vi "niRFSysCalReader Core.vi"(4 "Enable Interpolation?":bool, 6 "Power (dBm)":dbl, 7 "Frequency (Hz)":dbl, 8 "error in":errorcluster, 9 "niRFSysCalReader State":T1, 10 "Pathloss (dB)":dbl, 11 "niRFSysCalReader Handle":T2) -> (0 "error out":errorcluster, 2 "Pathloss (dB)":dbl, 3 "niRFSysCalReader Handle out":T2)   [LabVIEW 2016, in "niRFSysCalReader.lvlib"]
doc: "Core component of the niRFSysCalReader library."
uses:
  niRFSysCalReader.lvlib
  _INCLUDES/niRFSysCalReader Handle.ctl
  _INCLUDES/niRFSysCalReader Core States.ctl
  <vilib>/Utility/error.llb/Error Cluster From Error Code.vi
  <vilib>/ErrorRing/Error Ring.xnode
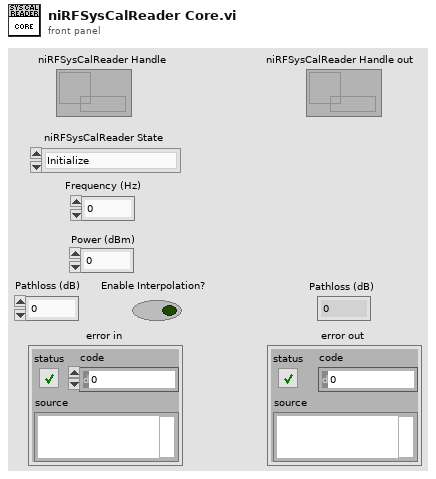
[diagram p1: front panel]
types:
  T1 = typedef "niRFSysCalReader.lvlib/niRFSysCalReader Core States.ctl" = enum16{"Initialize", "Interpolator State", "Add Pathloss", "Get Pathloss", "Remove Pathloss", "Close"}
  T2 = typedef "niRFSysCalReader.lvlib/niRFSysCalReader Handle.ctl" = refnum<data-value>
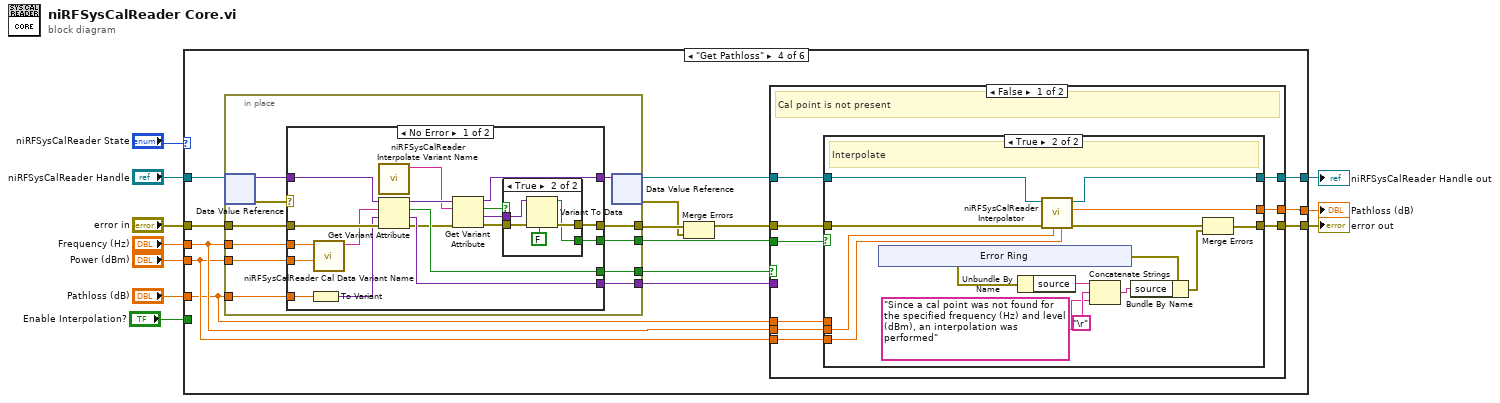
[diagram p0: block diagram]
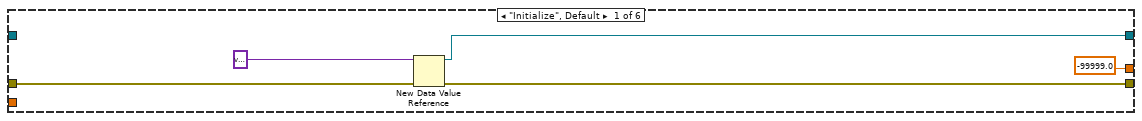
[diagram p2: hidden frame]
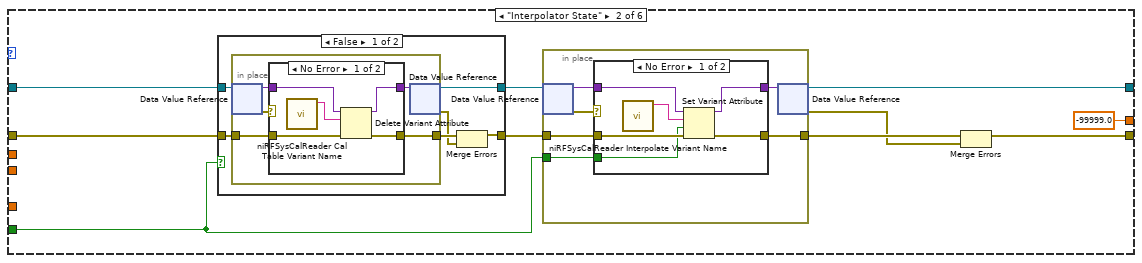
[diagram p3: hidden frame]
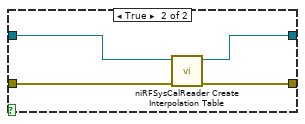
[diagram p5: hidden frame]
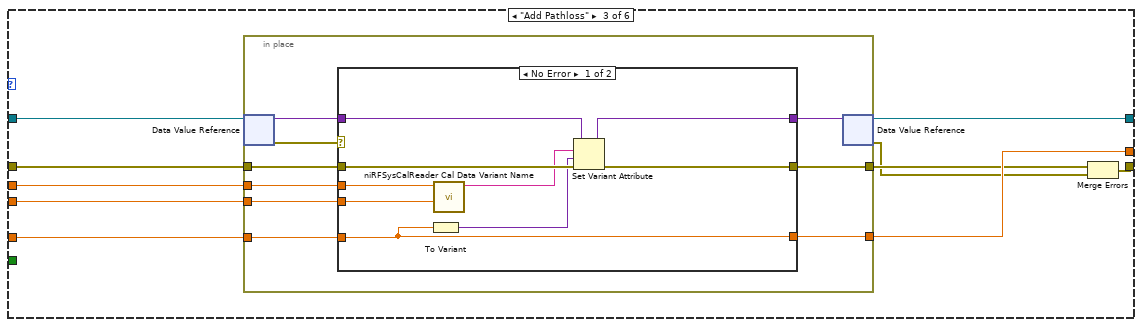
[diagram p7: hidden frame]
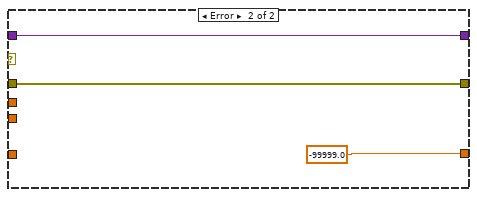
[diagram p8: hidden frame]
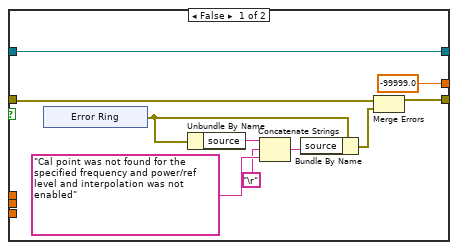
[diagram p9: hidden frame]
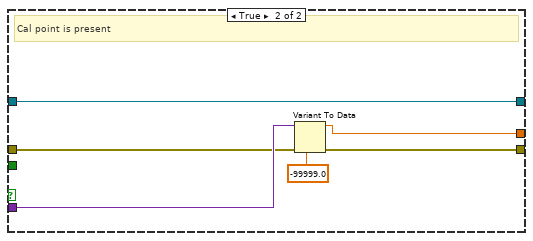
[diagram p10: hidden frame]
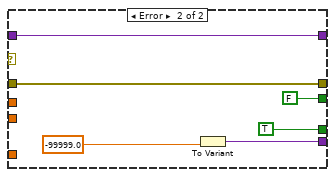
[diagram p12: hidden frame]
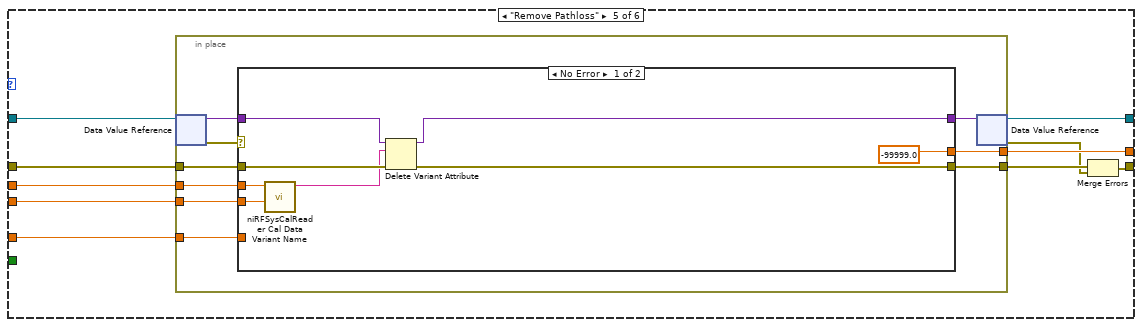
[diagram p13: hidden frame]
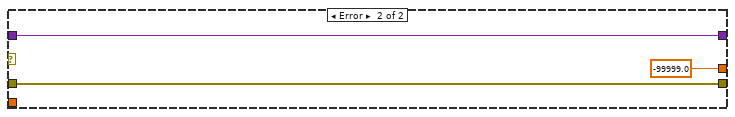
[diagram p14: hidden frame]
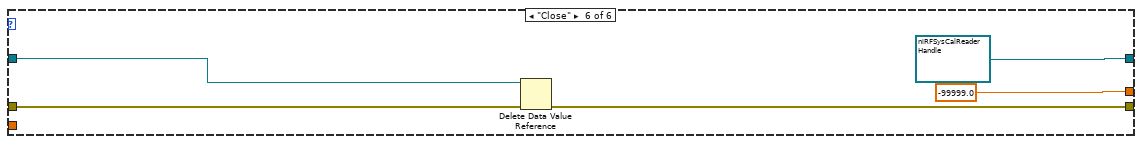
[diagram p15: hidden frame]
diagram:
  n1 = case shown="\"Get Pathloss\"" "niRFSysCalReader State" {
    tunnel: [w14 w25 w69 w97 w204 T2 refnum ("Cal Storage Handle in")] -> w3
    tunnel: [w13 w24 w68 w100 w203 w229] -> w2
    tunnel: "error in" -> [w12 w20 w70 w106 w205 w230]
    tunnel: "niRFSysCalReader Handle" -> [_ w22 w71 w107 w206 w231]
    tunnel: "Frequency (Hz)" -> [_ _ w67 w96 w202 _]
    tunnel: "Power (dBm)" -> [_ _ w66 w95 w201 _]
    tunnel: "Pathloss (dB)" -> [_ _ w65 w94 w200 _]
    tunnel: [-99999.0 -99999.0 ("Interpolated Pathloss (dB)") w64 w99 w199 -99999.0] -> w4
    tunnel: "Enable Interpolation?" -> [_ w16 _ _ _ _]
    frame "Initialize", Default {
      n2 = New Data Value Reference(data value=variant, error in=w12) -> (data value reference=w14:refnum<data-value>, error out=w13:errorcluster)
    }
    frame "Interpolator State" {
      n3 = case shown="False" w16 {
        tunnel: w22 -> [w31 w47]
        tunnel: [w30 w46] -> w21
        tunnel: w20 -> [w29 w45]
        tunnel: [w28 w44] -> w19
        frame False {
          n4 = in-place {
            in-place-border: w29 -> [w34]
            in-place-border: [w33] -> w27
            n5 = in-place-dvr #1(w31) -> (w36:variant, w32:errorcluster)
            n6 = case shown="No Error" w32 {
              tunnel: w36 -> [w41 w43]
              tunnel: [w40 w43] -> w35
              tunnel: w34 -> [w39 w42]
              tunnel: [w38 w42] -> w33
              frame No Error {
                n7 = call "niRFSysCalReader Cal Table Variant Name.vi"() -> ("Calibration Table Name"=w37:string)  [unwired: 11 in]
                n8 = Delete Variant Attribute(4:w39, 6:w37, 7:w41) -> (0:w38:errorcluster, 3:w40:variant)  [unwired: 1 out]
              }
              frame Error {
              }
            }
            n9 = in-place-dvr #1(w35) -> (w30:T2, w26:errorcluster)
          }
          n10 = Merge Errors(w27, w26) -> (w28:errorcluster)
        }
        frame True {
          n11 = call "niRFSysCalReader Create Interpolation Table.vi"("error in"=w45, "niRFSysCalReader Handle"=w47) -> ("error out"=w44:errorcluster, "niRFSysCalReader Handle out"=w46:T2)  [unwired: 7 in, 1 out]
        }
      }
      n12 = in-place {
        in-place-border: [w52] -> w18
        in-place-border: w19 -> [w50]
        in-place-border: w16 -> [w48]
        n13 = in-place-dvr #2(w21) -> (w53:variant, w49:errorcluster)
        n14 = case shown="No Error" w49 {
          tunnel: w53 -> [w59 w61]
          tunnel: [w57 w60] -> w52
          tunnel: [w56 w61] -> w51
          tunnel: w50 -> [w55 w60]
          tunnel: w48 -> [w54 _]
          frame No Error {
            n15 = call "niRFSysCalReader Interpolate Variant Name.vi"() -> ("Interpolation State Name"=w58:string)  [unwired: 11 in]
            n16 = Set Variant Attribute(Variant=w59, name=w58, value=w54, error in=w55) -> (Variant out=w56:variant, error out=w57:errorcluster)  [unwired: 1 out]
          }
          frame Error {
          }
        }
        n17 = in-place-dvr #2(w51) -> (w25:T2, w17:errorcluster)
      }
      n18 = Merge Errors(w18, w17) -> (w24:errorcluster)
    }
    frame "Add Pathloss" {
      n19 = in-place {
        in-place-border: w70 -> [w79]
        in-place-border: [w76] -> w63
        in-place-border: w67 -> [w75]
        in-place-border: w66 -> [w74]
        in-place-border: w65 -> [w73]
        in-place-border: [w72] -> w64
        n20 = in-place-dvr #3(w71) -> (w78:variant, w80:errorcluster)
        n21 = case shown="No Error" w80 {
          tunnel: w79 -> [w89 w91]
          tunnel: w78 -> [w84 w92]
          tunnel: [w83 w92] -> w77
          tunnel: [w88 w91] -> w76
          tunnel: w75 -> [w87 _]
          tunnel: w74 -> [w86 _]
          tunnel: w73 -> [w81 _]
          tunnel: [w81 -99999.0] -> w72
          frame No Error {
            n22 = To Variant(anything=w81) -> (Variant=w82:variant)
            n23 = call "niRFSysCalReader Cal Data Variant Name.vi"("Power (dBm)"=w86, "Frequency (Hz)"=w87) -> ("Calibration Data Name"=w85:string)  [unwired: 9 in]
            n24 = Set Variant Attribute(Variant=w84, name=w85, value=w82, error in=w89) -> (Variant out=w83:variant, error out=w88:errorcluster)  [unwired: 1 out]
          }
          frame Error {
          }
        }
        n25 = in-place-dvr #3(w77) -> (w69:T2, w62:errorcluster)
      }
      n26 = Merge Errors(w63, w62) -> (w68:errorcluster)
    }
    frame "Get Pathloss" {
      n27 = in-place {
        in-place-border: w106 -> [w164]
        in-place-border: [w161] -> w105
        in-place-border: w96 -> [w160]
        in-place-border: w95 -> [w159]
        in-place-border: w94 -> [w158]
        in-place-border: [w157] -> w103
        in-place-border: [w156] -> w102
        in-place-border: [w155] -> w93
        n28 = in-place-dvr #4(w107) -> (w163:variant, w165:errorcluster)
        n29 = case shown="No Error" w165 {
          tunnel: w164 -> [w183 w195]
          tunnel: w163 -> [w181 w196]
          tunnel: [w172 w196] -> w162
          tunnel: [w170 w195] -> w161
          tunnel: w160 -> [w178 _]
          tunnel: w159 -> [w177 _]
          tunnel: w158 -> [w180 _]
          tunnel: [w176 w192] -> w156
          tunnel: [w175 TRUE] -> w157
          tunnel: [w167 FALSE] -> w155
          frame No Error {
            n30 = To Variant(anything=w180) -> (Variant=w179:variant)
            n31 = call "niRFSysCalReader Cal Data Variant Name.vi"("Power (dBm)"=w177, "Frequency (Hz)"=w178) -> ("Calibration Data Name"=w182:string)  [unwired: 9 in]
            n32 = call "niRFSysCalReader Interpolate Variant Name.vi"() -> ("Interpolation State Name"=w166:string)  [unwired: 11 in]
            n33 = Get Variant Attribute(Variant=w181, name=w182, default value (empty Variant)=w179, error in=w183) -> (duplicate Variant=w173:variant, found=w175:bool, value=w176:variant, error out=w174:errorcluster)
            n34 = Get Variant Attribute(Variant=w173, name=w166, error in=w174) -> (duplicate Variant=w172:variant, found=w168:bool, value=w169:variant, error out=w171:errorcluster)  [unwired: 1 in]
            n35 = case shown="True" w168 {
              selector: w168 -> [w185 _]
              tunnel: w171 -> [w184 w190]
              tunnel: [w184 w189] -> w170
              tunnel: w169 -> [_ w188]
              tunnel: [w185 w186] -> w167
              frame False {
              }
              frame True {
                n36 = Variant To Data(error in=w190, type=FALSE, Variant=w188) -> (data=w186:bool, error out=w189:errorcluster)
              }
            }
          }
          frame Error {
            n37 = To Variant(anything=-99999.0) -> (Variant=w192:variant)
          }
        }
        n38 = in-place-dvr #4(w162) -> (w98:T2, w104:errorcluster)
      }
      n39 = Merge Errors(w105, w104) -> (w101:errorcluster)
      n40 = case shown="False" w103 {
        tunnel: [w116 w154] -> w100
        tunnel: [w115 w152] -> w99
        tunnel: w102 -> [_ w151]
        tunnel: w101 -> [w114 w150]
        tunnel: w98 -> [w113 w149]
        tunnel: [w112 w149] -> w97
        tunnel: w93 -> [w111 _]
        tunnel: w96 -> [w110 _]
        tunnel: w95 -> [w109 _]
        tunnel: w94 -> [w108 _]
        frame False {
          # "Cal point is not present"
          n41 = case shown="True" w111 {
            tunnel: [w123 w136] -> w116
            tunnel: [-99999.0 w144] -> w115
            tunnel: w114 -> [w124 w143]
            tunnel: w113 -> [w126 w142]
            tunnel: [w126 w141] -> w112
            tunnel: w110 -> [_ w132]
            tunnel: w109 -> [_ w131]
            tunnel: w108 -> [_ _]
            frame False {
              n42 = xnode "Error Ring"() -> ("error out"=w122:errorcluster)
              n43 = Unbundle By Name(w122) -> ("source"=w119:string)
              n44 = Concatenate Strings(w119, "\r", "Cal point was not found for the specified frequency and power/ref level and interpolation was not enabled" ("error message (\"\")")) -> (w118:string)
              n45 = Bundle By Name(cluster=w122, "source"=w118) -> (w117:errorcluster)
              n46 = Merge Errors(w124, w117) -> (w123:errorcluster)
            }
            frame True {
              # "Interpolate"
              n47 = xnode "Error Ring"() -> ("error out"=w133:errorcluster)
              n48 = Unbundle By Name(w133) -> ("source"=w139:string)
              n49 = call "niRFSysCalReader Interpolator.vi"("Power (dBm)"=w131, "Frequency (Hz)"=w132, "error in"=w143, "niRFSysCalReader Handle"=w142) -> ("error out"=w135:errorcluster, "Interpolated Pathloss (dB)"=w144:dbl, "niRFSysCalReader Handle out"=w141:T2)  [unwired: 5 in]
              n50 = Concatenate Strings(w139, "\r", "Since a cal point was not found for the specified frequency (Hz) and level (dBm), an interpolation was performed" ("error message (\"\")")) -> (w140:string)
              n51 = Bundle By Name(cluster=w133, "source"=w140) -> (w134:errorcluster)
              n52 = Merge Errors(w135, w134) -> (w136:errorcluster)
            }
          }
        }
        frame True {
          # "Cal point is present"
          n53 = Variant To Data(error in=w150, type=-99999.0, Variant=w151) -> (data=w152:dbl, error out=w154:errorcluster)
        }
      }
    }
    frame "Remove Pathloss" {
      n54 = in-place {
        in-place-border: w205 -> [w214]
        in-place-border: [w211] -> w198
        in-place-border: w202 -> [w210]
        in-place-border: w201 -> [w209]
        in-place-border: w200 -> [w208]
        in-place-border: [w207] -> w199
        n55 = in-place-dvr #5(w206) -> (w213:variant, w215:errorcluster)
        n56 = case shown="No Error" w215 {
          tunnel: w214 -> [w223 w225]
          tunnel: w213 -> [w219 w226]
          tunnel: [w218 w226] -> w212
          tunnel: [w220 w225] -> w211
          tunnel: w210 -> [w222 _]
          tunnel: w209 -> [w221 _]
          tunnel: w208 -> [_ _]
          tunnel: [-99999.0 -99999.0] -> w207
          frame No Error {
            n57 = call "niRFSysCalReader Cal Data Variant Name.vi"("Power (dBm)"=w221, "Frequency (Hz)"=w222) -> ("Calibration Data Name"=w217:string)  [unwired: 9 in]
            n58 = Delete Variant Attribute(4:w223, 6:w217, 7:w219) -> (0:w220:errorcluster, 3:w218:variant)  [unwired: 1 out]
          }
          frame Error {
          }
        }
        n59 = in-place-dvr #5(w212) -> (w204:T2, w197:errorcluster)
      }
      n60 = Merge Errors(w198, w197) -> (w203:errorcluster)
    }
    frame "Close" {
      n61 = Delete Data Value Reference(data value reference=w231, error in=w230) -> (error out=w229:errorcluster)  [unwired: 1 out]
    }
  }
  "Pathloss (dB)" <- w4
  "niRFSysCalReader Handle out" <- w3
  "error out" <- w2
